vi "Check_which_Conditions_are_met.vi"(8 "Error In":errorcluster, 10 "Settings cluster":T12 {"Calibration parameters"."True frame time, s" format="%.10g"; "Calibration parameters"."Disp. calibration info"."Speed, µl per ms" format="%.3g"; "Calibration parameters"."True FPS" format="%.10g"; "Calibration parameters"."Timing calibration sw/hw" format="%.10g"; "Conditions presets array"."Specifier(s)"."Validity criteria(s)"."Validity value" min=0.0 step=0.1 format="%.2g"; "Conditions presets array"."Specifier(s)"."Value" step=1.0 format="%#.2g"; "Recording and saving"."Data post-processing"."Order" min=3 max=11 step=2; "Recording and saving"."Data post-processing"."Length" min=5 max=301 step=2; "Geometry"."Cage diameter, mm" scale=0.0..340.0}, 11 "Current animal coordinates and stats":T9 {"Measurements and statistics"."Running, perc. of time" format="%05.2f"}) -> (0 "Error Out":errorcluster, 3 "Conditions are TRUE":bool[](array[boolean]), 5 "Conditions presets array out":T1 {"Specifier(s)"."Validity criteria(s)"."Validity value" min=0.0 step=0.1 format="%.2g"; "Specifier(s)"."Value" step=1.0 format="%#.2g"}, 7 "IO parameters.IO inversion config.":u16)   [LabVIEW 2018, in "TTL IO.lvlib"]
uses:
  TTL IO.lvlib
  SubVi's/Controls/CTL_Settings_cluster.ctl
  SubVi's/Controls/CTL_Histogram_parameters.ctl
  SubVi's/Controls/CTL_Filter_selector.ctl
  SubVi's/Controls/CTL_Acquisition_speed_selector.ctl
  SubVi's/Controls/CTL_Segmented_plot_parameters.ctl
  SubVi's/Controls/CTL_IO_params_cluster.ctl
  SubVi's/Controls/CTL_Conditions_Array.ctl
  SubVi's/Controls/CTL_Conditions_Cluster.ctl
  SubVi's/Controls/CTL_Condition_type.ctl
  SubVi's/Controls/CTL_Comparison_type.ctl
  SubVi's/Controls/CTL_Validity_check_criteria.ctl
  SubVi's/Controls/CTL_Response_info.ctl
  SubVi's/Controls/CTL_Condition_response_type.ctl
  SubVi's/Controls/CTL_Reponse_port_info.ctl
  SubVi's/Controls/CTL_Calibration_parameters.ctl
  SubVi's/Controls/CTL_Dispenser_calibration_info.ctl
  SubVi's/Controls/CTL_Full_data_frame.ctl
  SubVi's/Controls/CTL_Animal_Coordinates_and_Speed.ctl
  SubVi's/Controls/CTL_Measurements_and_Statistics.ctl
  Common_Resources.lvlib
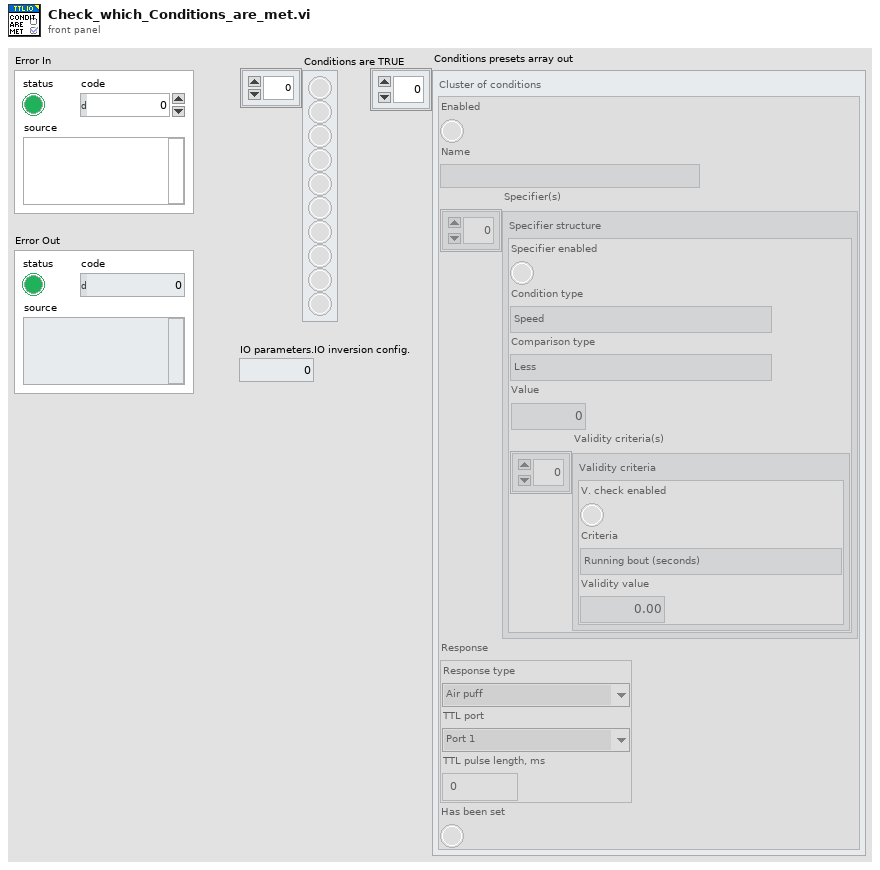
[diagram p1: front panel]
types:
  T1 = typedef "Common_Resources.lvlib/CTL_Conditions_Array.ctl" = T2[]
  T2 = typedef "Common_Resources.lvlib/CTL_Conditions_Cluster.ctl" = cluster{"Enabled":bool, "Name":string, "Specifier(s)":cluster{"Specifier enabled":bool, "Condition type":T3, "Comparison type":T4, "Value":dbl, "Validity criteria(s)":cluster{"V. check enabled":bool, "Criteria":T5, "Validity value":dbl}[]}[], "Response":T6, "Has been set":bool}
  T3 = typedef "Common_Resources.lvlib/CTL_Condition_type.ctl" = enum16{"Speed", "Zone", "Angle to wall"}
  T4 = typedef "Common_Resources.lvlib/CTL_Comparison_type.ctl" = enum16{"Less", "Less or Equal", "Equal", "Greater or Equal", "Greater", "Not Equal"}
  T5 = typedef "Common_Resources.lvlib/CTL_Validity_check_criteria.ctl" = enum16{"Running bout (seconds)", "Running bout (meters)"}
  T6 = typedef "Common_Resources.lvlib/CTL_Response_info.ctl" = cluster{"Response type":T7, "TTL port":T8, "TTL pulse length, ms":dbl}
  T7 = typedef "Common_Resources.lvlib/CTL_Condition_response_type.ctl" = enum16{"None", "Air puff", "Liquid reward"}
  T8 = typedef "Common_Resources.lvlib/CTL_Reponse_port_info.ctl" = enum16{"Port 1", "Port 2", "Port 3", "Port 4"}
  T9 = typedef "Common_Resources.lvlib/CTL_Full_data_frame.ctl" = cluster{"Times":cluster{"ms since ON":u32, "delta time":u32, "Frame timestamp":timestamp}, "TTLs":cluster{"TTL input":i16, "TTL output":i16}, "Animal coordinates":T10, "Magnets coords raw":cluster{"X1 raw":dbl, "Y1 raw":dbl, "X2 raw":dbl, "Y2 raw":dbl}, "Measurements and statistics":T11}
  T10 = typedef "Common_Resources.lvlib/CTL_Animal_Coordinates_and_Speed.ctl" = cluster{"R from center":dbl, "phi (mouse angular position in the cage)":dbl, "alpha (mouse rot. angle)":dbl, "X":dbl, "Y":dbl, "theta (from center towards mouse)":dbl, "beta (cage rot. against mouse)":dbl, "w (mouse angle to wall)":dbl, "Speed (filtered)":dbl}
  T11 = typedef "Common_Resources.lvlib/CTL_Measurements_and_Statistics.ctl" = cluster{"Zone #":i8, "Histogram":dbl[], "Running, perc. of time":dbl, "Run, meters":dbl, "Avg. speed":dbl}
  T12 = typedef "Common_Resources.lvlib/CTL_Settings_cluster.ctl" = cluster{"Defaults":cluster{"Default User":dbl, "VISA Resource Name ":string, "Histogram parameters":T13}, "Recording and saving":cluster{"Researcher name":string, "Name prefix":string, "Data post-processing":T14, "Stop at":dbl, "\"Stop at\" enabled":bool, "Default save folder path":path, "Acquisition FPS":T15}, "Geometry":T16, "IO parameters":T17, "Conditions presets array":T1, "Calibration parameters":T18, "Settings loaded OK":bool}
  T13 = typedef "Common_Resources.lvlib/CTL_Histogram_parameters.ctl" = cluster{"max":dbl, "min":dbl, "# bins":i32, "threshold":dbl, "thr. type":enum16{"higher accepted", "lower accepted"}}
  T14 = typedef "Common_Resources.lvlib/CTL_Filter_selector.ctl" = cluster{"Filter type":enum16{"None", "Savitzky-Golay"}, "Length":i32, "Order":i32}
  T15 = typedef "Common_Resources.lvlib/CTL_Acquisition_speed_selector.ctl" = enum16{"Max", "Optimal", "Eco"}
  T16 = typedef "Common_Resources.lvlib/CTL_Segmented_plot_parameters.ctl" = cluster{"Cage diameter, mm":u16, "Starting angle MIDFIELD":i16, "Starting angle BORDER":i16, "Radius, mm CENTER":u16, "Radius, mm MIDFIELD":u16, "N segments MIDFIELD":u8, "N segments BORDER":u8, "R-gap, mm":sgl, "Bridge swap":bool, "Bridge H. offset":sgl, "Bridge V. offset":sgl, "Twisted neck":bool, "Alt. magn. orientation":bool, "Sensor board size":enum16{"Small", "Large"}}
  T17 = typedef "Common_Resources.lvlib/CTL_IO_params_cluster.ctl" = cluster{"IO general config.":u16, "IO 1 configuration":u16, "IO 2 configuration":u16, "IO 3 configuration":u16, "IO 4 configuration":u16, "Activate ext. RS-232":u16, "IO inversion config.":u16, "Sync capability":u8}
  T18 = typedef "Common_Resources.lvlib/CTL_Calibration_parameters.ctl" = cluster{"Timing calibration sw/hw":dbl, "True FPS":dbl, "True frame time, s":dbl, "Disp. calibration info":T19}
  T19 = typedef "Common_Resources.lvlib/CTL_Dispenser_calibration_info.ctl" = cluster{"Channel":u8, "Speed, µl per ms":dbl}[]
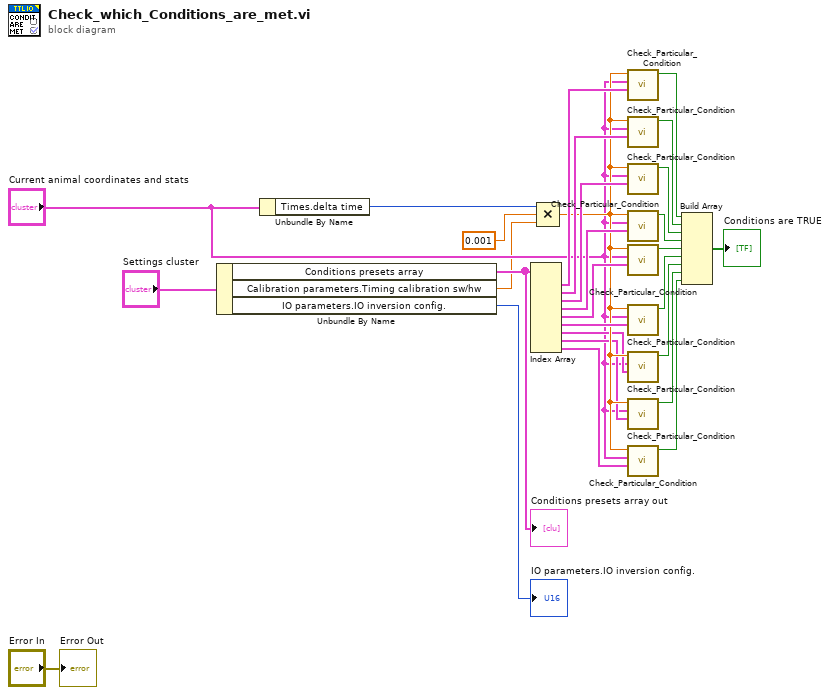
[diagram p0: block diagram]
diagram:
  n1 = Unbundle By Name("Settings cluster") -> ("Conditions presets array"=w26:T1, "Calibration parameters.Timing calibration sw/hw"=w2:dbl, "IO parameters.IO inversion config."=→"IO parameters.IO inversion config.":u16)
  "Conditions presets array out" <- w26
  n2 = Unbundle By Name("Current animal coordinates and stats") -> ("Times.delta time"=w25:u32)
  n3 = Index Array(array=w26) -> (element #1=w24:T2, element #2=w23:T2, element #3=w18:T2, element #4=w17:T2, element #5=w16:T2, element #6=w15:T2, element #7=w9:T2, element #8=w8:T2, element #9=w7:T2)  [unwired: 9 in]
  n4 = Compound Arithmetic op=MULTIPLY(w25, 0.001 ("y"), w2) -> (w10:dbl)
  n5 = call "Check_Particular_Condition.vi"("Cluster of conditions"=w24, "Current animal coordinates and stats"="Current animal coordinates and stats", "Frame length, ms"=w10) -> ("Condition is met"=w21:bool)  [unwired: 7 in, 1 out]
  n6 = call "Check_Particular_Condition.vi"("Cluster of conditions"=w23, "Current animal coordinates and stats"="Current animal coordinates and stats", "Frame length, ms"=w10) -> ("Condition is met"=w22:bool)  [unwired: 7 in, 1 out]
  n7 = call "Check_Particular_Condition.vi"("Cluster of conditions"=w18, "Current animal coordinates and stats"="Current animal coordinates and stats", "Frame length, ms"=w10) -> ("Condition is met"=w14:bool)  [unwired: 7 in, 1 out]
  n8 = call "Check_Particular_Condition.vi"("Cluster of conditions"=w17, "Current animal coordinates and stats"="Current animal coordinates and stats", "Frame length, ms"=w10) -> ("Condition is met"=w13:bool)  [unwired: 7 in, 1 out]
  n9 = call "Check_Particular_Condition.vi"("Cluster of conditions"=w16, "Current animal coordinates and stats"="Current animal coordinates and stats", "Frame length, ms"=w10) -> ("Condition is met"=w12:bool)  [unwired: 7 in, 1 out]
  n10 = call "Check_Particular_Condition.vi"("Cluster of conditions"=w15, "Current animal coordinates and stats"="Current animal coordinates and stats", "Frame length, ms"=w10) -> ("Condition is met"=w11:bool)  [unwired: 7 in, 1 out]
  n11 = call "Check_Particular_Condition.vi"("Cluster of conditions"=w9, "Current animal coordinates and stats"="Current animal coordinates and stats", "Frame length, ms"=w10) -> ("Condition is met"=w5:bool)  [unwired: 7 in, 1 out]
  n12 = call "Check_Particular_Condition.vi"("Cluster of conditions"=w8, "Current animal coordinates and stats"="Current animal coordinates and stats", "Frame length, ms"=w10) -> ("Condition is met"=w4:bool)  [unwired: 7 in, 1 out]
  n13 = call "Check_Particular_Condition.vi"("Cluster of conditions"=w7, "Current animal coordinates and stats"="Current animal coordinates and stats", "Frame length, ms"=w10) -> ("Condition is met"=w3:bool)  [unwired: 7 in, 1 out]
  n14 = Build Array(w21, w22, w14, w13, w12, w11, w5, w4, w3) -> (→"Conditions are TRUE":bool[])
  "Error Out" <- "Error In"
